vi "Write topic.vi"(8 "error in (no error)":errorcluster, 10 "topic":string, 11 "SingleTopic in":refnum<class "SingleTopic.lvclass">) -> (0 "error out":errorcluster, 3 "SingleTopic out":refnum<class "SingleTopic.lvclass">)   [LabVIEW 2023, in "uLib.lvlib" / "SingleTopic.lvclass"]
uses:
  SingleTopic.lvclass
  SingleTopic.lvclass/SingleTopic.ctl
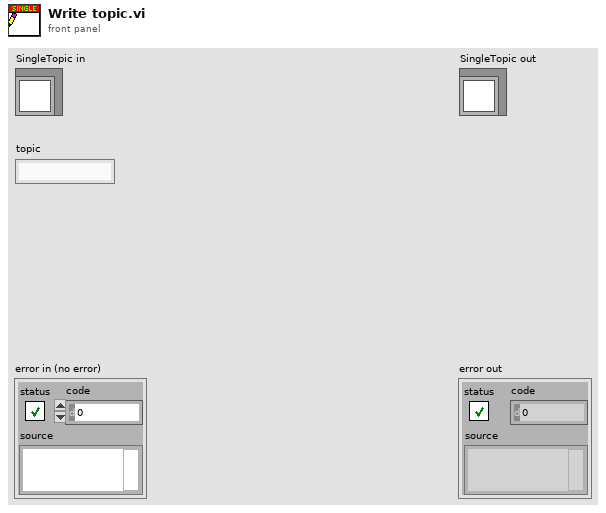
[diagram p1: front panel]
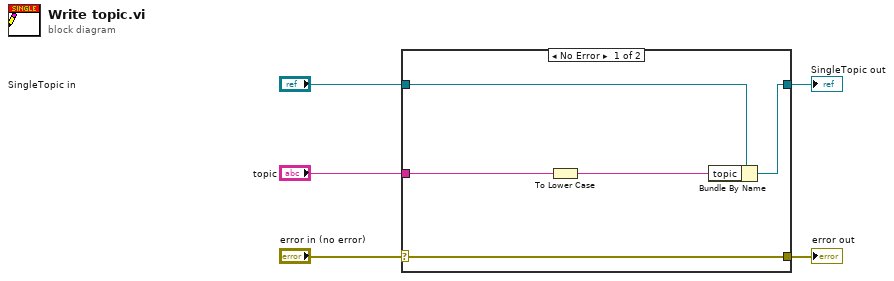
[diagram p0: block diagram]
diagram:
  n1 = case shown="No Error" "error in (no error)" {
    selector: "error in (no error)" -> [w10 w11]
    tunnel: [w10 w11] -> w4
    tunnel: [w8 w12] -> w2
    tunnel: "SingleTopic in" -> [w9 w12]
    tunnel: "topic" -> [w7 _]
    frame No Error {
      n2 = To Lower Case(string=w7) -> (all lower case string=w6:string)
      n3 = Bundle By Name(cluster=w9, "topic"=w6) -> (w8:refnum<class "SingleTopic.lvclass">)
    }
    frame Error {
    }
  }
  "error out" <- w4
  "SingleTopic out" <- w2
